vi "lab8_vi1.vi"() -> ()   [LabVIEW 2020]
uses:
  <vilib>/Platform/TimedLoop/XDataNode/timing_clust.ctl
  <vilib>/Platform/TimedLoop/XDataNode/nitl_modes.ctl
  <vilib>/Platform/TimedLoop/XDataNode/wakeup.ctl
  <vilib>/Platform/TimedLoop/scheduler/LVUserAPI/_suppVIs/Create_1kHz_TSource.vi
  <vilib>/platform/TimedLoop/XDataNode/XDataNode.xnode
  <vilib>/Platform/TimedLoop/XDataNode/XDNodeRunTimeDep.lvlib
panel:
  in  "Synchronizacja":bool
  out "Koniec 2":bool
  out "Error 2":errorcluster
  out "L2 Stop":dbl
  out "L2 End":i64
  out "Nr pêtli 2":i64
  out "L1 Stop":dbl
  out "czas_pocz":u32
  out "Koniec 1":bool
  out "Error 1":errorcluster
  out "Nr pêtli 1":i64
  out "L1 End":i64
  in  "Okres [s]":dbl=5.0 min=0.5 max=20.0 step=0.5
  out "S0 End":i64
  out "S0 Start":i64
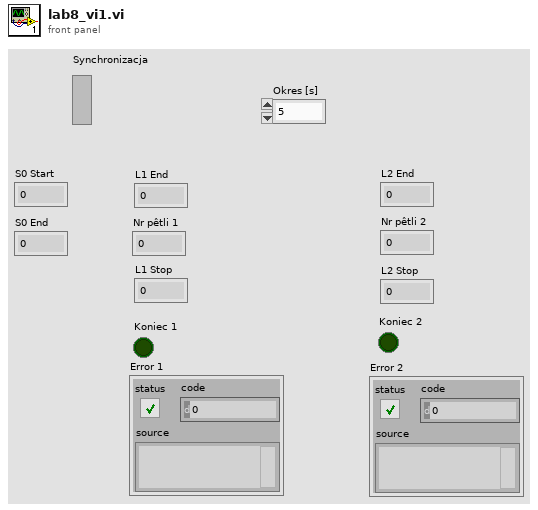
[diagram p1: front panel]
types:
  T1 = typedef "XDNodeRunTimeDep.lvlib/timing_clust.ctl" = cluster{"Expected End [f-1]":u64, "Actual End [f-1]":u64, "Finished Late? [f-1]":bool, "Expected End [i-1]":u64, "Actual End [i-1]":u64, "Finished Late? [i-1]":bool, "Expected Start [i]":u64, "Actual Start [i]":u64, "Expected Start [f]":u64, "Actual Start [f]":u64, "Source Name":string, "Structure Name":string, "Period":i64, "Deadline":i64, "Offset":i64, "Start":i64, "Priority":i32, "Timeout":i32, "Mode":T2, "Wakeup Reason":T3, "Error":errorcluster, "Source Type":string, "Secondary Source Type":string, "Global End Time":u64, "Global Start Time":u64, "Frame Duration":u64, "Iteration Duration":u64, "Assigned CPU":i32, "I/O Scan Engine Mode":u32}
  T2 = typedef "XDNodeRunTimeDep.lvlib/nitl_modes.ctl" = enum32{"No Change", "Process missed periods, maintain original phase", "Discard missed periods, maintain original phase", "Process missed periods, ignore original phase", "Discard missed periods, ignore original phase"}
  T3 = typedef "XDNodeRunTimeDep.lvlib/wakeup.ctl" = enum32{"Normal", "Aborted", "Asynchronous wakeup", "Timing source error", "Timed loop error", "Timeout"}
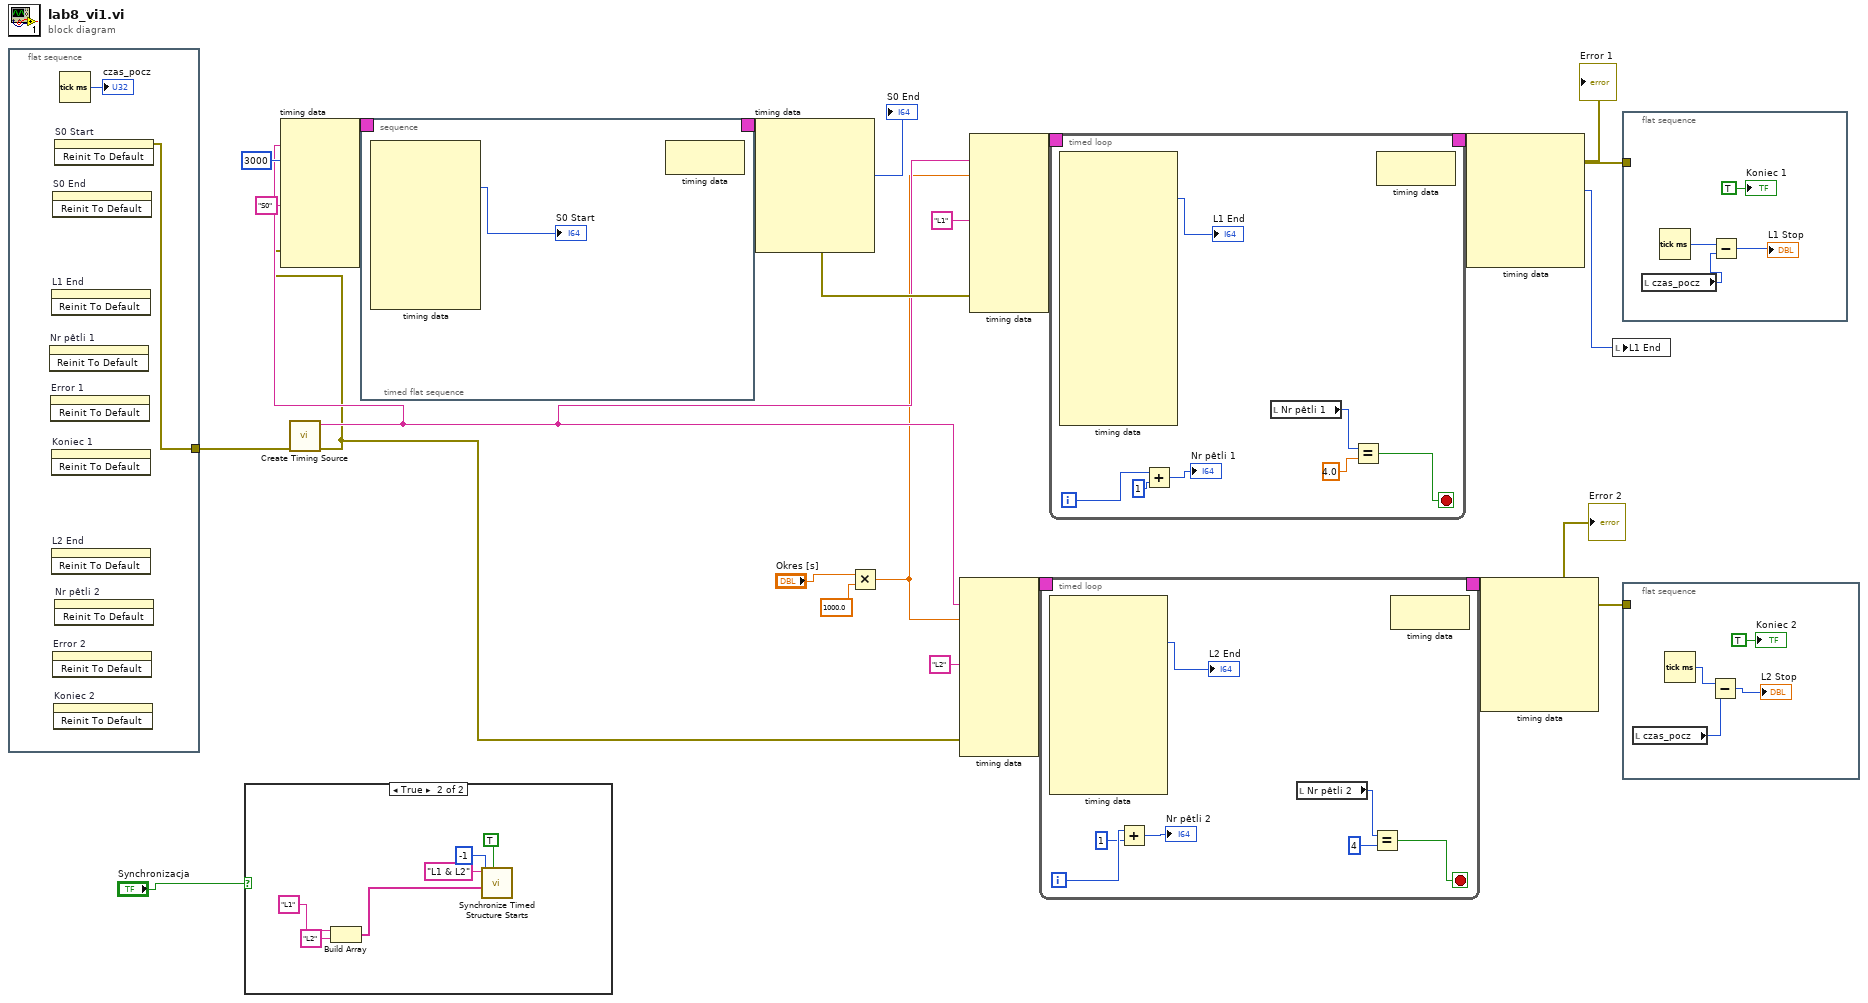
[diagram p0: block diagram]
diagram:
  n1 = flat-sequence {
    tunnel: [w23] -> w2
    frame #0 {
      n2 = invoke on="Nr pêtli 1" class="DigNum (strict)" method="Reinit To Default"() -> ()  [unwired: 3 in, 3 out]
      n3 = invoke on="Error 1" class="Clust (strict)" method="Reinit To Default"() -> ()  [unwired: 3 in, 3 out]
      n4 = invoke on="L1 End" class="DigNum (strict)" method="Reinit To Default"() -> ()  [unwired: 3 in, 3 out]
      n5 = invoke on="Koniec 1" class="Bool (strict)" method="Reinit To Default"() -> ()  [unwired: 3 in, 3 out]
      n6 = invoke on="L2 End" class="DigNum (strict)" method="Reinit To Default"() -> ()  [unwired: 3 in, 3 out]
      n7 = invoke on="S0 End" class="DigNum (strict)" method="Reinit To Default"() -> ()  [unwired: 3 in, 3 out]
      n8 = invoke on="Error 2" class="Clust (strict)" method="Reinit To Default"() -> ()  [unwired: 3 in, 3 out]
      n9 = invoke on="Koniec 2" class="Bool (strict)" method="Reinit To Default"() -> ()  [unwired: 3 in, 3 out]
      n10 = invoke on="S0 Start" class="DigNum (strict)" method="Reinit To Default"() -> (error out=w23:errorcluster)  [unwired: 3 in, 2 out]
      n11 = invoke on="Nr pêtli 2" class="DigNum (strict)" method="Reinit To Default"() -> ()  [unwired: 3 in, 3 out]
      n12 = Tick Count (ms)() -> (millisecond timer value=→"czas_pocz":u32)
    }
  }
  n13 = case shown="True" "Synchronizacja" {
    frame False {
    }
    frame True {
      n14 = Build Array("L1", "L2" ("element")) -> (w25:string[])
      n15 = call <vilib>:"Synchronize Timed Structure Starts.vi"("replace (T)"=TRUE, "timed structure names"=w25, "timeout ms (10000)"=-1, "synchronization group name"="L1 & L2") -> ()  [unwired: 6 in, 2 out]
    }
  }
  n16 = call-poly <vilib>:"Create Timing Source.vi"("error in (no error)"=w2) -> ("error out"=w4:errorcluster, "name (out)"=w6:string)  [unwired: 9 in]
  n17 = node-c288(w6, i64 3000 ("Offset"), "S0" ("Structure Name"), w4) -> (w22:T1)  [unwired: 4 in]
  n18 = timed-sequence {
    timing: w22 -> [_]
    timing-out: [_] -> w21
    n19 = timed-flat-sequence {
      n20 = node-c288() -> (→"S0 Start":i64)  [unwired: 1 in, 9 out]
      n21 = node-c288() -> ()  [unwired: 1 in, 1 out]
    }
  }
  n22 = node-c288(w21) -> (w18:errorcluster, →"S0 End":i64)  [unwired: 5 out]
  n23 = Multiply(x="Okres [s]", y=1000.0) -> (x*y=w5:dbl)
  n24 = node-c288(w6, w5, "L2" ("Structure Name"), w4) -> (w9:T1)  [unwired: 6 in]
  n25 = node-c288(w6, w5, "L1" ("Structure Name"), w18) -> (w20:T1)  [unwired: 6 in]
  n26 = timed-loop {
    timing: w9 -> [_]
    timing-out: [_] -> w8
    i -> [w41]
    stop <- w36 stop-if-true
    n27 = node-c288() -> (→"L2 End":i64)  [unwired: 1 in, 11 out]
    n28 = Add(x=w41, y=1) -> (x+y=→"Nr pêtli 2":i32)
    n29 = local read "Nr pêtli 2"() -> (w38:i64)
    n30 = Equal?(x=w38, y=i64 4) -> (x = y?=w36:bool)
    n31 = node-c288() -> ()  [unwired: 1 in, 1 out]
  }
  n32 = timed-loop {
    timing: w20 -> [_]
    timing-out: [_] -> w19
    i -> [w50]
    stop <- w45 stop-if-true
    n33 = node-c288() -> (→"L1 End":i64)  [unwired: 1 in, 16 out]
    n34 = Add(x=w50, y=1) -> (x+y=→"Nr pêtli 1":i32)
    n35 = local read "Nr pêtli 1"() -> (w47:i64)
    n36 = Equal?(x=w47, y=4.0) -> (x = y?=w45:bool)
    n37 = node-c288() -> ()  [unwired: 1 in, 1 out]
  }
  n38 = node-c288(w19) -> (w17:errorcluster, w10:i64)  [unwired: 5 out]
  "Error 1" <- w17
  n39 = node-c288(w8) -> (w3:errorcluster)  [unwired: 6 out]
  "Error 2" <- w3
  n40 = local write "L1 End"(w10) -> ()
  n41 = flat-sequence {
    tunnel: w17 -> [_]
    frame #0 {
      n42 = local read "czas_pocz"() -> (w55:u32)
      n43 = Tick Count (ms)() -> (millisecond timer value=w56:u32)
      n44 = Subtract(x=w56, y=w55) -> (x-y=→"L1 Stop":u32)
      "Koniec 1" <- TRUE ("Koniec 1")
    }
  }
  n45 = flat-sequence {
    tunnel: w3 -> [_]
    frame #0 {
      n46 = local read "czas_pocz"() -> (w61:u32)
      n47 = Tick Count (ms)() -> (millisecond timer value=w62:u32)
      n48 = Subtract(x=w62, y=w61) -> (x-y=→"L2 Stop":u32)
      "Koniec 2" <- TRUE ("Koniec 2")
    }
  }
